vi "BuildTags.vi"(8 "error in (no error)":errorcluster, 11 "Menu in":refnum<class "MGI_Menu.lvclass">) -> (0 "error out":errorcluster, 3 "Menu out":refnum<class "MGI_Menu.lvclass">)   [LabVIEW 2016, in "MGI_Menu.lvclass"]
doc: "Builds the full tags (recursively) of the menu items.\n\nAuthored by Derek E. Trepanier\nsupport@mooregoodideas.com\nwww.mooregoodideas.com\n\nCopyright (c) 2012, Moore Good Ideas, Inc.\n\nAll rights reserved.\n\nRedistribution and use in source and binary forms, with or without modification, are permitted provided that the following conditions are met:\n\n * Redistributions of source code must retain the above copyright notice, this list of conditions and the following disclaimer.\n * Redistributions in binary form must reproduce the above copyright notice, this list of conditions and the following disclaimer in the documentation and/or other materials provided with the distribution.\n * Neither the name of Moore Good Ideas, Inc. nor the names of its contributors may be used to endorse or promote products derived from this software without specific prior written permission.\n\nTHIS SOFTWARE IS PROVIDED BY THE COPYRIGHT HOLDERS AND CONTRIBUTORS \"AS IS\" AND ANY EXPRESS OR IMPLIED WARRANTIES, INCLUDING, BUT NOT LIMITED TO, THE IMPLIED WARRANTIES OF MERCHANTABILITY AND FITNESS FOR A PARTICULAR PURPOSE ARE DISCLAIMED. IN NO EVENT SHALL THE COPYRIGHT OWNER OR CONTRIBUTORS BE LIABLE FOR ANY DIRECT, INDIRECT, INCIDENTAL, SPECIAL, EXEMPLARY, OR CONSEQUENTIAL DAMAGES (INCLUDING, BUT NOT LIMITED TO, PROCUREMENT OF SUBSTITUTE GOODS OR SERVICES; LOSS OF USE, DATA, OR PROFITS; OR BUSINESS INTERRUPTION) HOWEVER CAUSED AND ON ANY THEORY OF LIABILITY, WHETHER IN CONTRACT, STRICT LIABILITY, OR TORT (INCLUDING NEGLIGENCE OR OTHERWISE) ARISING IN ANY WAY OUT OF THE USE OF THIS SOFTWARE, EVEN IF ADVISED OF THE POSSIBILITY OF SUCH DAMAGE."
uses:
  <userlib>/_MGI/Menu Building/MenuTypes/MGI_Menu.lvclass
  <userlib>/_MGI/Menu Building/MenuTypes/MGI_Menu.lvclass/MGI_Menu.ctl
  <userlib>/_MGI/Menu Building/MenuItem/MGI_MenuItem.lvclass
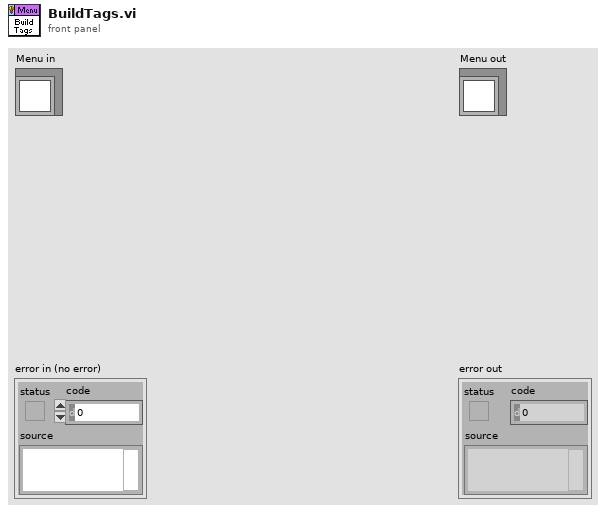
[diagram p1: front panel]
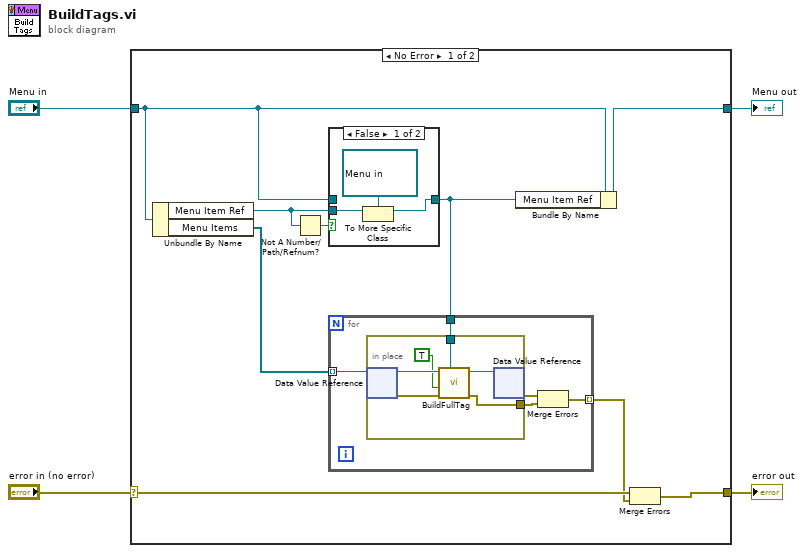
[diagram p0: block diagram]
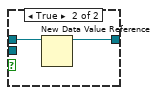
[diagram p2: hidden frame]
diagram:
  n1 = case shown="No Error" "error in (no error)" {
    selector: "error in (no error)" -> [w13 w31]
    tunnel: [w11 w31] -> w3
    tunnel: [w8 w30] -> w1
    tunnel: "Menu in" -> [w9 w30]
    frame No Error {
      n2 = Unbundle By Name(w9) -> ("Menu Item Ref"=w5:refnum<data-value>, "Menu Items"=w12:refnum<data-value>[])
      n3 = Not A Number/Path/Refnum?(number/path/refnum=w5) -> (NaN/Path/Refnum?=w6:bool)
      n4 = case shown="False" w6 {
        tunnel: w9 -> [_ w18]
        tunnel: [w15 w17] -> w7
        tunnel: w5 -> [w16 _]
        frame False {
          n5 = To More Specific Class(target class=refnum<data-value> refnum, reference=w16) -> (specific class reference=w15:refnum<data-value>)  [unwired: 1 in, 1 out]
        }
        frame True {
          n6 = New Data Value Reference(data value=w18) -> (data value reference=w17:refnum<data-value>)  [unwired: 1 in, 1 out]
        }
      }
      n7 = for {
        tunnel: w12 -> [w23] mode=indexing
        tunnel: [w21] -> w10 mode=indexing
        tunnel: w7 -> [w19]
        n8 = in-place {
          in-place-border: [w25] -> w20
          in-place-border: w19 -> [w24]
          n9 = in-place-dvr #1(w23) -> (w29:refnum<class "MGI_MenuItem.lvclass">, w26:errorcluster)
          n10 = call <userlib>:"BuildFullTag.vi"("Menu Ref"=w24, "error in (no error)"=w26, "Build Full Tree"=TRUE, "MGI_MenuItem in"=w29) -> ("error out"=w25:errorcluster, "MGI_MenuItem out"=w28:refnum<class "MGI_MenuItem.lvclass">)  [unwired: 6 in]
          n11 = in-place-dvr #1(w28) -> (w22:errorcluster)  [unwired: 1 out]
        }
        n12 = Merge Errors(w22, w20) -> (w21:errorcluster)
      }
      n13 = Bundle By Name(cluster=w9, "Menu Item Ref"=w7) -> (w8:refnum<class "MGI_Menu.lvclass">)
      n14 = Merge Errors(w13, w10) -> (w11:errorcluster)
    }
    frame Error {
    }
  }
  "error out" <- w3
  "Menu out" <- w1
